vi "1_Power_Transmission_Line_Fault_Classification(Training).vi"() -> ()   [LabVIEW 2020]
uses:
  <vilib>/Ngene/DeepLTK/Toolkit/NN_Train/Controls/NN_LR_Policy_Cfg.ctl
  <vilib>/Ngene/DeepLTK/Toolkit/NN_Train/Controls/NN_LR_Policy_Type.ctl
  <vilib>/Ngene/DeepLTK/Toolkit/NN_Train/Controls/NN_Train_Session_Data.ctl
  <vilib>/Ngene/DeepLTK/Toolkit/NN_Train/Controls/NN_Train_Params.ctl
  <vilib>/Ngene/DeepLTK/Toolkit/NN_Train/Controls/NN_Train_Optimizer.ctl
  <vilib>/Ngene/DeepLTK/Toolkit/NN_Train/Controls/NN_Train_Data_Sampling.ctl
  <vilib>/Ngene/DeepLTK/Toolkit/NN_Network/Controls/NN_Device.ctl
  <vilib>/Ngene/DeepLTK/Toolkit/NN_Layers/Layers/Input/Controls/NN_Layer_Config(Input1D).ctl
  <vilib>/Ngene/DeepLTK/Toolkit/NN_Layers/Layers/FC/Controls/NN_Layer_Config(FC).ctl
  <vilib>/Ngene/DeepLTK/Toolkit/NN_Activations/Controls/NN_Activation_Type.ctl
  <vilib>/Ngene/DeepLTK/Toolkit/NN_Layers/Controls/NN_Layer_Init_Params.ctl
  <vilib>/Ngene/DeepLTK/Toolkit/NN_Layers/Controls/NN_Layer_Weight_Init_Type.ctl
  <vilib>/Ngene/DeepLTK/Toolkit/NN_Network/Controls/NN_Save_Before_Destroy_Options.ctl
  <vilib>/Ngene/DeepLTK/Toolkit/NN_Layers/Layers/DropOut3D/Controls/NN_Layer_Config(DropOut3D).ctl
  <vilib>/Ngene/DeepLTK/Toolkit/NN_Layers/Layers/Input/NN_Layer_Create(Input1D).vi
  <vilib>/Ngene/DeepLTK/Toolkit/NN_Layers/Layers/FC/NN_Layer_Create(FC).vi
  <vilib>/Ngene/DeepLTK/Toolkit/NN_Layers/Layers/Dropout/NN_Layer_Create(DropOut).vi
  <vilib>/Ngene/DeepLTK/Toolkit/NN_Layers/Layers/SoftMax/NN_Layer_Create(SoftMax).vi
  <vilib>/Ngene/DeepLTK/Toolkit/NN_Train/Loss_Functions/NN_Set_Loss(CrossEntropy).vi
  <vilib>/Ngene/DeepLTK/Toolkit/NN_Network/subVIs/NN_Predict/NN_Predict(In1D_Out1D).vi
  <vilib>/Ngene/DeepLTK/Toolkit/NN_Train/Eval_Loss/NN_Eval_Test_Error_Loss/NN_Eval(In1D_Out1D).vi
  <vilib>/Ngene/DeepLTK/Toolkit/NN_Train/Eval_Loss/NN_Calc_Cofusion_Matrix/NN_Calc_Confusion_Matrix(In1D_Out1D).vi
  <vilib>/Ngene/DeepLTK/Toolkit/Deep_Learning_Toolkit_by_Ngene.lvlib
  <vilib>/ptbypt/NI_PtbyPt.lvlib
panel:
  in  "Tab Control":enum32{"Training", "Evaluation"}(tab)
  in  "LR Update Policy":T1={"Policy_Type"=enum."Step", "LR0"=0.0001, "k"=30.0, "WarmUp_Policy"=enum."Ramp", "WarmUp_Iter"=1000, "WarmUp_Ratio"=10.0} {"WarmUp_Ratio" min=1; "WarmUp_Iter" min=1; "LR0" format="%.7f"}
  out "Session Data":T3={"Epochs"=141.0176, "Tot_Iter"=33051, "LR"=6.25e-06, "LR_iter"=33052} {"LR" format="%#_3g"}
  in  "NN_Train_Params":T4={"Optimizer"=enum."Adam", "Beta_1"=0.9, "Beta_2"=0.999, "Weight Decay(L1)"=7e-07, "Weight Decay(L2)"=7e-07, "Data_Sampling"=enum."Random"}
  in  "Stop Training":bool
  out "Test Error":sgl=0.021 format="%#.6g"
  out "Test Loss":sgl=0.07218283 format="%#.6g"
  in  "NN_Device":T7=enum."GPU"
  out "Loss Graphs":cluster{"mean":dbl, "mean":dbl, "mean":dbl}(graph)={"mean"=0.09143101282417775, "mean"=0.07218282669782639, "mean"=0.020999999716877937}
  in  "Eval":bool
  out "Training Loss":sgl=0.04577865 format="%#.6g"
  in  "Train dataset path":path=path "D:/Ngene/GitHub/deepltk_examples/2_Waveform_Processing/23_Power_Transmission_Line_Fault_Classification/Dataset/Train"
  in  "Test dataset path":path=path "D:/Ngene/GitHub/deepltk_examples/2_Waveform_Processing/23_Power_Transmission_Line_Fault_Classification/Dataset/Test"
  out "Time_Elapsed":dbl=146.3093000000008 format="%<%H:%M:%S>t"
  out "Confusion Matrix":string[][](table)=[["1500", "0", "0", "0", "0", "0", "1.0000"], ["0", "1499", "0", "1", "0", "0", "0.9993"], ["0", "0", "1496", "0", "0", "4", "0.9973"], ["0", "0", "0", "1404", "94", "2", "0.9360"], ["0", "0", "0", "49", "1449", "2", "0.9660"], ["0", "0", "36", "1", "0", "1463", "0.9753"], ["1.0000", "1.0000", "0.9765", "0.9649", "0.9391", "0.9946", ""]]
  # "Overview: This example demonstrating the usage of Deep Learning Toolkit for solving  Power Transmission Line Fault classification problem.\nRequirements: Deep Learning Toolkit for LabVIEW\nInstructions:\n1.  Run the VI with current configuration of the training parameters and Learning Rate update policy\n2. Observe how the training loss is decreasing\n3. Wait about 2 minutes and press the \"Stop\" button when the loss is not decreasing anymore."
  # "Power Transmission Line Fault Classification - Training"
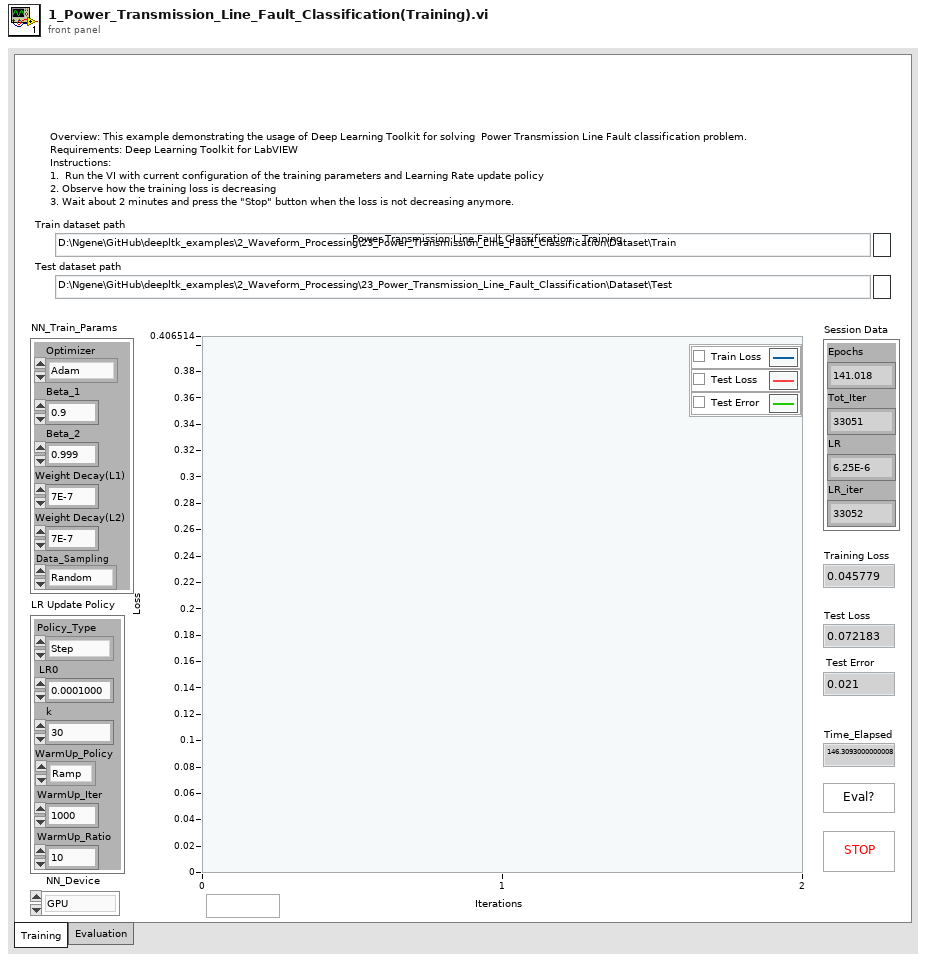
[diagram p1: front panel]
types:
  T1 = typedef "Deep_Learning_Toolkit_by_Ngene.lvlib/NN_LR_Policy_Cfg.ctl" = cluster{"Policy_Type":T2, "LR0":dbl, "k":sgl, "WarmUp_Policy":enum16{"Step", "Ramp"}, "WarmUp_Iter":i32, "WarmUp_Ratio":sgl}
  T2 = typedef "Deep_Learning_Toolkit_by_Ngene.lvlib/NN_LR_Policy_Type.ctl" = enum16{"Manual", "Step", "Exp", "1/t"}
  T3 = typedef "Deep_Learning_Toolkit_by_Ngene.lvlib/NN_Train_Session_Data.ctl" = cluster{"Epochs":sgl, "Tot_Iter":i32, "LR":sgl, "LR_iter":i32}
  T4 = typedef "Deep_Learning_Toolkit_by_Ngene.lvlib/NN_Train_Params.ctl" = cluster{"Optimizer":T5, "Beta_1":sgl, "Beta_2":sgl, "Weight Decay(L1)":sgl, "Weight Decay(L2)":sgl, "Data_Sampling":T6}
  T5 = typedef "Deep_Learning_Toolkit_by_Ngene.lvlib/NN_Train_Optimizer.ctl" = enum16{"SGD", "Adam", "Adagrad", "Adadelta", "RMSProp", "Nesterov"}
  T6 = typedef "Deep_Learning_Toolkit_by_Ngene.lvlib/NN_Train_Data_Sampling.ctl" = enum16{"Random", "Sequential"}
  T7 = typedef "Deep_Learning_Toolkit_by_Ngene.lvlib/NN_Device.ctl" = enum16{"CPU", "GPU"}
  T8 = typedef "Deep_Learning_Toolkit_by_Ngene.lvlib/NN_Layer_Config(DropOut3D).ctl" = cluster{"Name":string, "Probability":sgl}
  T9 = typedef "Deep_Learning_Toolkit_by_Ngene.lvlib/NN_Save_Before_Destroy_Options.ctl" = cluster{"CFG?":bool, "Weights?":bool, "Render?":bool}
  T10 = typedef "Deep_Learning_Toolkit_by_Ngene.lvlib/NN_Layer_Config(FC).ctl" = cluster{"Name":string, "Size":i32, "BN":bool, "Activation":T11, "Init_Params":T12, "Custom_Params":string}
  T11 = typedef "Deep_Learning_Toolkit_by_Ngene.lvlib/NN_Activation_Type.ctl" = enum16{"Sigmoid", "ReLU", "LReLU", "ReLU6", "tanh", "Swish", "Mish", "None"}
  T12 = typedef "Deep_Learning_Toolkit_by_Ngene.lvlib/NN_Layer_Init_Params.ctl" = cluster{"Init_Type":T13, "Value":sgl}
  T13 = typedef "Deep_Learning_Toolkit_by_Ngene.lvlib/NN_Layer_Weight_Init_Type.ctl" = enum16{"Const", "Uniform", "Gaussian", "Xavier"}
  T14 = typedef "Deep_Learning_Toolkit_by_Ngene.lvlib/NN_Layer_Config(Input1D).ctl" = cluster{"Name":string, "Size":i32}
  T15 = typedef "Deep_Learning_Toolkit_by_Ngene.lvlib/NN_DataSets_All(In1D_Out1D).ctl" = cluster{"Train":T16, "Validation":T16, "Test":T16}
  T16 = typedef "Deep_Learning_Toolkit_by_Ngene.lvlib/NN_DataSet(In1D_Out1D).ctl" = cluster{"Inputs Ref.":T17, "Outputs Ref.":T17, "Dims_In":i32, "Dataset_Size":i32, "Outputs_idx Ref.":T18, "Dims_Out":i32, "Labels":string[], "File Paths":path[]}
  T17 = typedef "Deep_Learning_Toolkit_by_Ngene.lvlib/NN_Data_ref(2D_SGL).ctl" = refnum<data-value>
  T18 = typedef "Deep_Learning_Toolkit_by_Ngene.lvlib/NN_Data_ref(1D_I32).ctl" = refnum<data-value>
  T19 = typedef "Deep_Learning_Toolkit_by_Ngene.lvlib/NN.ctl" = cluster{"Name":string, "No of Layers":i32, "mBatch":i32, "Layers":T20[], "Dimty":T21, "Dims_In":T22, "Dims_Out":T22, "Working_Dir":path, "Train?":bool, "Train_Params":T4, "LR_Update_Policy":T1, "Session Data":T3, "Ground_truth":T23, "NNg_hdls":T24, "NN_Device":T7, "GPU Id":i32, "Labels":string[], "Receptive Field":T25[], "Loss_Type":T26, "Loss_Cfg_Prms":variant}
  T20 = typedef "Deep_Learning_Toolkit_by_Ngene.lvlib/NN_Layer_ref.ctl" = refnum<data-value>
  T21 = typedef "Deep_Learning_Toolkit_by_Ngene.lvlib/NN_In_Out_Dim-ty.ctl" = enum8{"In1D_Out1D", "In3D_Out1D", "In3D_Out3D", "In3D_OutBBox"}
  T22 = typedef "Deep_Learning_Toolkit_by_Ngene.lvlib/NN_Dims(C,H,W).ctl" = cluster{"C":i32, "H":i32, "W":i32}
  T23 = typedef "Deep_Learning_Toolkit_by_Ngene.lvlib/NN_Ground_truth.ctl" = cluster{"Y":variant, "Y_idx":T18}
  T24 = typedef "Deep_Learning_Toolkit_by_Ngene.lvlib/nng_cuda_handles.ctl" = cluster{"cudnn":u64, "cublas":u64, "stream":u64, "curand":u64}
  T25 = typedef "Deep_Learning_Toolkit_by_Ngene.lvlib/NN_Dims(V,H).ctl" = cluster{"V":i32, "H":i32}
  T26 = typedef "Deep_Learning_Toolkit_by_Ngene.lvlib/NN_Loss_Type.ctl" = enum16{"None", "MSE", "CrossEntropy", "YOLO_v2"}
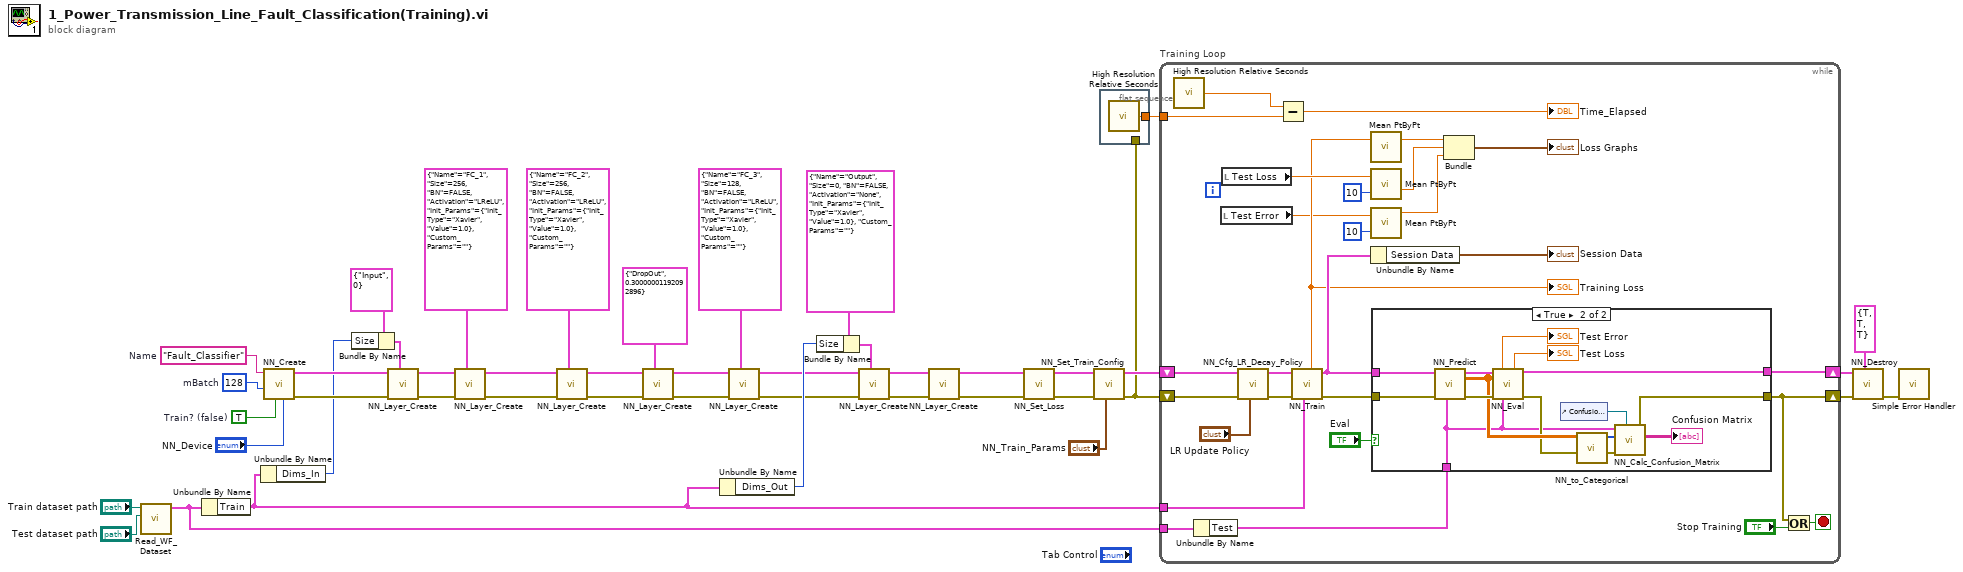
[diagram p0: block diagram]
diagram:
  w27 = "Fault_Classifier"  # Name
  w28 = 128  # mBatch
  w29 = TRUE  # Train? (false)
  n1 = call "Read_WF_Dataset.vi"("Test dataset path"="Test dataset path", "Train dataset path"="Train dataset path") -> ("NN_Dataset"=w11:T15)  [unwired: 9 in]
  n2 = Unbundle By Name(w11) -> ("Train"=w12:T16)
  n3 = Unbundle By Name(w12) -> ("Dims_In"=w13:i32)
  n4 = call <vilib>:"NN_Create.vi"("NN_Device"="NN_Device", "Train? (false)"=w29, "mBatch (1)"=w28, "Name"=w27) -> ("error out"=w43:errorcluster, "NN out"=w44:T19)  [unwired: 6 in]
  n5 = Bundle By Name(cluster=T14 {"Name"="Input", "Size"=0} ("Input1D_Cfg"), "Size"=w13) -> (w35:T14)
  n6 = call-poly <vilib>:"NN_Layer_Create.vi"("Input1D_Cfg"=w35, "error in (no error)"=w43, "NN in"=w44) -> ("error out"=w31:errorcluster, "NN out"=w32:T19)  [unwired: 6 in, 1 out]
  n7 = call-poly <vilib>:"NN_Layer_Create.vi"("FC_Cfg"=T10 {"Name"="FC_1", "Size"=256, "BN"=FALSE, "Activation"=enum."LReLU", "Init_Params"={"Init_Type"=enum."Xavier", "Value"=1.0}, "Custom_Params"=""} ("FC_Cfg_1"), "error in (no error)"=w31, "NN in"=w32) -> ("error out"=w2:errorcluster, "NN out"=w3:T19)  [unwired: 6 in, 1 out]
  n8 = call-poly <vilib>:"NN_Layer_Create.vi"("FC_Cfg"=T10 {"Name"="FC_2", "Size"=256, "BN"=FALSE, "Activation"=enum."LReLU", "Init_Params"={"Init_Type"=enum."Xavier", "Value"=1.0}, "Custom_Params"=""} ("FC_Cfg_1"), "error in (no error)"=w2, "NN in"=w3) -> ("error out"=w4:errorcluster, "NN out"=w7:T19)  [unwired: 6 in, 1 out]
  n9 = call-poly <vilib>:"NN_Layer_Create.vi"("DropOut_Cfg"=T8 {"Name"="DropOut", "Probability"=0.3}, "error in (no error)"=w4, "NN in"=w7) -> ("error out"=w5:errorcluster, "NN out"=w6:T19)  [unwired: 6 in, 1 out]
  n10 = Unbundle By Name(w12) -> ("Dims_Out"=w33:i32)
  n11 = call-poly <vilib>:"NN_Layer_Create.vi"("FC_Cfg"=T10 {"Name"="FC_3", "Size"=128, "BN"=FALSE, "Activation"=enum."LReLU", "Init_Params"={"Init_Type"=enum."Xavier", "Value"=1.0}, "Custom_Params"=""} ("FC_Cfg_1"), "error in (no error)"=w5, "NN in"=w6) -> ("error out"=w18:errorcluster, "NN out"=w19:T19)  [unwired: 6 in, 1 out]
  n12 = Bundle By Name(cluster=T10 {"Name"="Output", "Size"=0, "BN"=FALSE, "Activation"=enum."None", "Init_Params"={"Init_Type"=enum."Xavier", "Value"=1.0}, "Custom_Params"=""} ("FC_Cfg_1"), "Size"=w33) -> (w34:T10)
  n13 = call-poly <vilib>:"NN_Layer_Create.vi"("FC_Cfg"=w34, "error in (no error)"=w18, "NN in"=w19) -> ("error out"=w38:errorcluster, "NN out"=w39:T19)  [unwired: 6 in, 1 out]
  n14 = call-poly <vilib>:"NN_Layer_Create.vi"("error in (no error)"=w38, "NN in"=w39) -> ("error out"=w24:errorcluster, "NN out"=w40:T19)  [unwired: 7 in, 1 out]
  n15 = call-poly <vilib>:"NN_Set_Loss.vi"("error in (no error)"=w24, "NN in"=w40) -> ("error out"=w23:errorcluster, "NN out"=w25:T19)  [unwired: 8 in]
  n16 = call <vilib>:"NN_Set_Train_Config.vi"("NN_Train_Params"="NN_Train_Params", "error in (no error)"=w23, "NN in"=w25) -> ("error out"=w9:errorcluster, "NN out"=w30:T19)  [unwired: 7 in]
  n17 = flat-sequence {
    tunnel: w9 -> [_]
    tunnel: [w45] -> w8
    frame #0 {
      n18 = call <vilib>:"High Resolution Relative Seconds.vi"() -> ("relative seconds"=w45:dbl)
    }
  }
  n19 = while "Training Loop" {
    shift-right: [w58] -> w16
    shift-left: w9 -> [w68]
    shift-right: [w64] -> w17
    shift-left: w30 -> [w71]
    tunnel: w12 -> [w53]
    tunnel: w11 -> [w54]
    tunnel: w8 -> [w51]
    stop <- w59 stop-if-true
    n20 = call <vilib>:"High Resolution Relative Seconds.vi"() -> ("relative seconds"=w50:dbl)
    n21 = Unbundle By Name(w54) -> ("Test"=w52:T16)
    n22 = local read "Test Error"() -> (w47:sgl)
    n23 = local read "Test Loss"() -> (w62:sgl)
    n24 = call <vilib>:"NN_Cfg_LR_Decay_Policy.vi"("LR_Decay_Params"="LR Update Policy", "error in (no error)"=w68, "NN in"=w71) -> ("error out"=w69:errorcluster, "NN out"=w70:T19)  [unwired: 7 in]
    n25 = Subtract(x=w50, y=w51) -> (x-y=→"Time_Elapsed":dbl)
    n26 = call <vilib>:"NN_Train.vi"("Train Dataset"=w53, "error in (no error)"=w69, "NN in"=w70) -> ("error out"=w65:errorcluster, "NN out"=w66:T19, "Loss"=w60:sgl)  [unwired: 5 in, 1 out]
    "Training Loss" <- w60
    n27 = call <vilib>:"Mean PtByPt.vi"("x"=w60) -> ("mean"=w56:dbl)  [unwired: 3 in, 1 out]
    n28 = call <vilib>:"Mean PtByPt.vi"("x"=w62, "sample length"=10) -> ("mean"=w57:dbl)  [unwired: 2 in, 1 out]
    n29 = call <vilib>:"Mean PtByPt.vi"("x"=w47, "sample length"=10) -> ("mean"=w46:dbl)  [unwired: 2 in, 1 out]
    n30 = Unbundle By Name(w66) -> ("Session Data"=→"Session Data":T3)
    n31 = case shown="True" "Eval" {
      tunnel: w66 -> [w75 w88]
      tunnel: w65 -> [w74 w87]
      tunnel: [w75 w86] -> w64
      tunnel: [w74 w79] -> w58
      tunnel: w52 -> [_ w76]
      frame False {
      }
      frame True {
        n32 = call-poly <vilib>:"NN_Predict.vi"("Dataset"=w76, "error in (no error)"=w87, "NN in"=w88) -> ("error out"=w89:errorcluster, "Predictions"=w82:sgl[][], "NN out"=w83:T19)  [unwired: 6 in]
        n33 = call-poly <vilib>:"NN_Eval.vi"("NN in"=w83, "Predictions"=w82, "error in (no error)"=w89, "Dataset"=w76) -> ("Error"=→"Test Error":sgl, "Loss"=→"Test Loss":sgl, "NN out"=w86:T19, "error out"=w80:errorcluster)  [unwired: 7 in, 1 out]
        n34 = control-ref of="Confusion Matrix"() -> (w77:refnum<vi>)
        n35 = call <vilib>:"NN_to_Categorical.vi"("Prediction"=w82) -> ("Label_Idx"=w81:i32[])  [unwired: 10 in]
        n36 = call-poly <vilib>:"NN_Calc_Confusion_Matrix.vi"("Confusion Matrix (Table) ref."=w77, "error in (no error)"=w80, "Predictions"=w81, "Dataset"=w76) -> ("error out"=w79:errorcluster, "Confusion Matrix (Table)"=→"Confusion Matrix":string[][])  [unwired: 3 in, 3 out]
      }
    }
    n37 = Bundle("mean"=w56, "mean"=w57, "mean"=w46) -> (→"Loss Graphs":cluster{"mean":dbl, "mean":dbl, "mean":dbl})  [unwired: 1 in]
    n38 = Or(x=w58, y="Stop Training") -> (x .or. y?=w59:bool)
  }
  n39 = call <vilib>:"NN_Destroy.vi"("Save (T, T, T)"=T9 {"CFG?"=TRUE, "Weights?"=TRUE, "Render?"=TRUE}, "error in (no error)"=w16, "NN in"=w17) -> ("error out"=w37:errorcluster)  [unwired: 8 in]
  n40 = call <vilib>:"Simple Error Handler.vi"("error in (no error)"=w37) -> ()  [unwired: 4 in, 5 out]
